vi "high speed voltage.vi"() -> ()   [LabVIEW 2018]
uses:
  <vilib>/DAQmx/read.llb/DAQmx Read (Analog 2D DBL NChan NSamp).vi
  <vilib>/DAQmx/create/channels.llb/DAQmx Create Channel (AI-Pressure-Bridge-Two-Point-Linear).vi
  <vilib>/DAQmx/configure/timing.llb/DAQmx Timing (Sample Clock).vi
  <vilib>/DAQmx/miscellaneous.llb/DAQmx Fill In Error Info.vi
panel:
  out "data 2":dbl[][](array[numeric]) format="%0.2f"
  in  "STOP":bool
  out "data":dbl[][](array[numeric]) format="%0.2f"
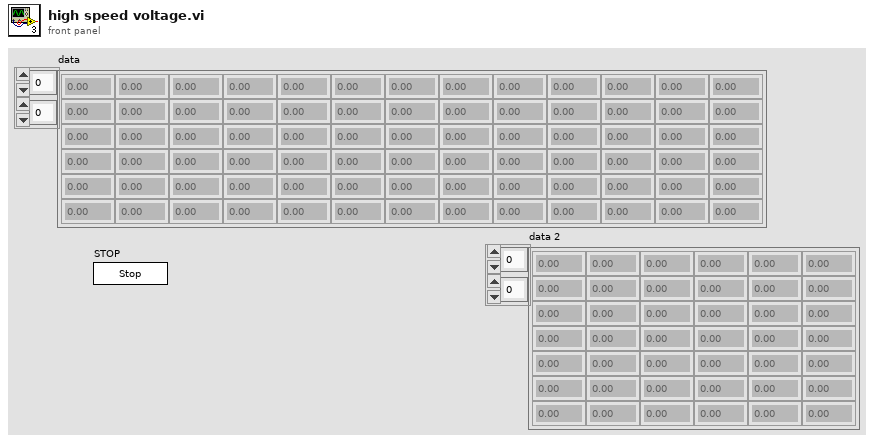
[diagram p1: front panel]
types:
  T1 = cluster{"first electrical value":dbl, "second electrical value":dbl, "electrical units":i32, "first physical value":dbl, "second physical value":dbl, "physical units":i32}
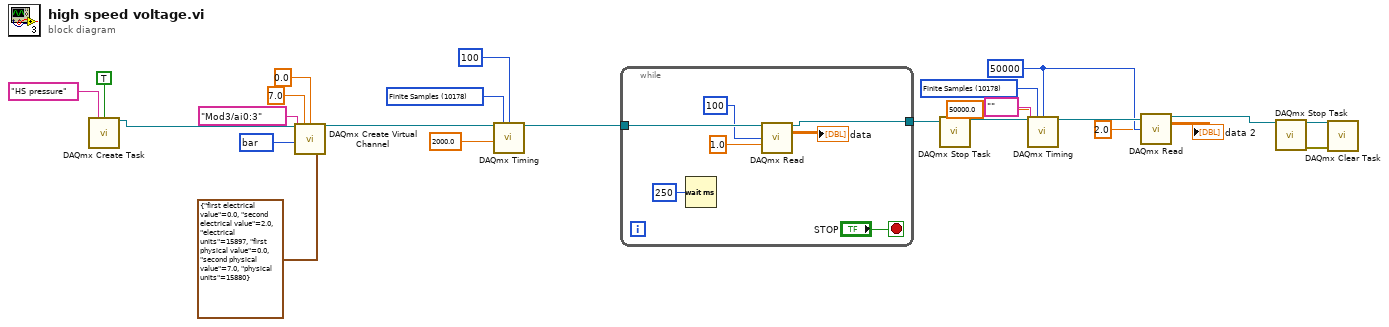
[diagram p0: block diagram]
diagram:
  w6 = 50000 ("samples per channel")
  w9 = 10178 items=["Finite Samples"=10178, "Continuous Samples"=10123, "Hardware Timed Single Point"=12522] ("sample mode")
  w16 = 10178 items=["Finite Samples"=10178, "Continuous Samples"=10123, "Hardware Timed Single Point"=12522] ("sample mode")
  w18 = 15880 items=["Pascals"=10081, "psi"=15879, "bar"=15880, "From Custom Scale"=10065] ("units")
  n1 = call <vilib>:"DAQmx Create Task.vi"("new task name"="HS pressure", "auto cleanup"=TRUE) -> ("task out"=w24:refnum<k21>)  [unwired: 12 in, 1 out]
  n2 = call-poly <vilib>:"DAQmx Create Virtual Channel.vi"("task in"=w24, "maximum value"=7.0, "minimum value"=0.0, "physical channels"=tag "Mod3/ai0:3", "units"=w18, "scaling information"=T1 {"first electrical value"=0.0, "second electrical value"=2.0, "electrical units"=15897, "first physical value"=0.0, "second physical value"=7.0, "physical units"=15880}) -> ("task out"=w17:refnum<k21>)  [unwired: 8 in, 1 out]
  n3 = call-poly <vilib>:"DAQmx Timing.vi"("task/channels in"=w17, "sample mode"=w16, "samples per channel"=100, "rate"=2000.0) -> ("task out"=w13:refnum<k21>)  [unwired: 10 in, 1 out]
  n4 = while {
    tunnel: w13 -> [w31]
    tunnel: [w27] -> w12
    stop <- "STOP" stop-if-true
    n5 = Wait (ms)(milliseconds to wait=u32 250) -> ()  [unwired: 1 out]
    n6 = call-poly <vilib>:"DAQmx Read.vi"("task/channels in"=w31, "number of samples per channel"=100, "timeout"=1.0) -> ("task out"=w27:refnum<k21>, "data"=→"data":dbl[][])  [unwired: 10 in, 1 out]
  }
  n7 = call <vilib>:"DAQmx Stop Task.vi"("task/channels in"=w12) -> ("task out"=w11:refnum<k21>)  [unwired: 13 in, 1 out]
  n8 = call-poly <vilib>:"DAQmx Timing.vi"("task/channels in"=w11, "sample mode"=w9, "samples per channel"=w6, "rate"=50000.0, "source"=tag "") -> ("task out"=w7:refnum<k21>)  [unwired: 9 in, 1 out]
  n9 = call-poly <vilib>:"DAQmx Read.vi"("task/channels in"=w7, "number of samples per channel"=w6, "timeout"=2.0) -> ("task out"=w3:refnum<k21>, "data"=→"data 2":dbl[][])  [unwired: 10 in, 1 out]
  n10 = call <vilib>:"DAQmx Stop Task.vi"("task/channels in"=w3) -> ("task out"=w2:refnum<k21>, "error out"=w1:errorcluster)  [unwired: 13 in]
  n11 = call <vilib>:"DAQmx Clear Task.vi"("task in"=w2, "error in"=w1) -> ()  [unwired: 13 in, 1 out]
